vi "Read Connected String.vi"(8 "error in (no error)":errorcluster, 11 "DataBase_SQL in":refnum<class "DataBase_SQL.lvclass">) -> (0 "error out":errorcluster, 2 "Connected String":string, 3 "DataBase_SQL out":refnum<class "DataBase_SQL.lvclass">)   [LabVIEW 2021, in "DataBase_SQL.lvclass"]
uses:
  <userlib>/John_Lib/DataBase/DataBase_SQL/DataBase_SQL.lvclass
  <userlib>/John_Lib/DataBase/DataBase_SQL/DataBase_SQL.lvclass/DataBase_SQL.ctl
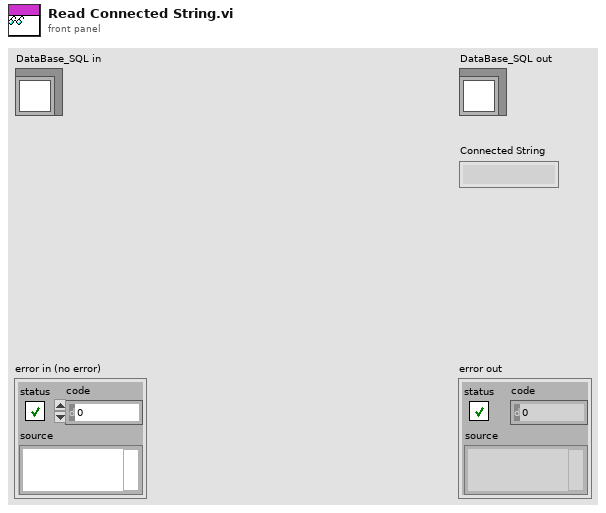
[diagram p1: front panel]
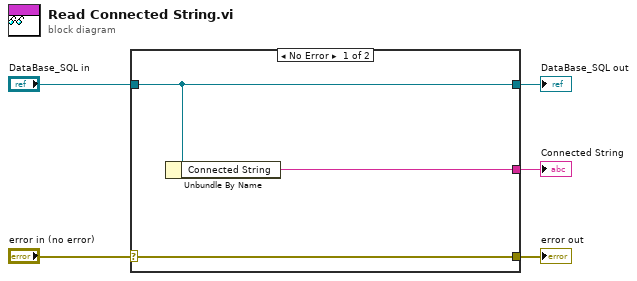
[diagram p0: block diagram]
diagram:
  n1 = case shown="No Error" "error in (no error)" {
    selector: "error in (no error)" -> [w8 w9]
    tunnel: [w8 w9] -> w4
    tunnel: [w7 w10] -> w2
    tunnel: "DataBase_SQL in" -> [w7 w10]
    tunnel: [w6 _] -> w1
    frame No Error {
      n2 = Unbundle By Name(w7) -> ("Connected String"=w6:string)
    }
    frame Error {
    }
  }
  "error out" <- w4
  "DataBase_SQL out" <- w2
  "Connected String" <- w1
